vi "HEWH Draw Initialize All Parameters.vi"(0 "Core HEWH Data Input in":T1 {"Test Patten Setup"."PRAT/RLT Sequence"."Time" format="%<%H:%M:%S>t"; "Test Patten Setup"."Total Gallons Schedule" format="%.2f"}, 1 "Station Draw Info":T3 {"Time" format="%<%H:%M:%S>t"}, 2 "Skip Draw":bool, 3 "Skip Purge":bool, 5 "Error In":errorcluster, 7 "K-Factor (Intellifaucet)":dbl, 9 "Current Cond":T8, 11 "K-Factor (Flow)":dbl, 13 "Intellifaucet Type":string) -> (14 "Core HEWH Data Input out":T1 {"Test Patten Setup"."PRAT/RLT Sequence"."Time" format="%<%H:%M:%S>t"; "Test Patten Setup"."Total Gallons Schedule" format="%.2f"}, 15 "Skip Draw":bool, 16 "Skip Purge":bool, 17 "Skip Valve Setup":bool, 19 "Error Out":errorcluster)   [LabVIEW 2016]
uses:
  Type Definitions/HEWH Special Condition Check.ctl
  Type Definitions/HEWH Output Information.ctl
  Type Definitions/HEWH Draw Pattern Setup.ctl
  Type Definitions/PRAT Test.ctl
  Utility/Save File/File Setup (Public)/Type Definition/Save File HEWH Heating Control Mode.ctl
  Type Definitions/Terminate Draw Conditions.ctl
  Type Definitions/HEWH Start Conditions.ctl
  Type Definitions/Check Special Condtions.ctl
  Type Definitions/HEWH Draw Flag ENUM.ctl
  Type Definitions/HEWH Specific DAQ.ctl
  Type Definitions/HEWH Power Data.ctl
  Type Definitions/HEWH Power Elements.ctl
  Utility/Type Definitions/UTILITY Power Analyzer.ctl
  Type Definitions/HEWH Calc and Calibration.ctl
  Utility/Save File/File Setup (Public)/Type Definition/Save File DOE LabView Program.ctl
  Custom Instrument Control/MW100/Type Definitions/Station ID Selector.ctl
  Range/Type Definitions/RANGE ANSI Rate.ctl
  Utility/Save File/File Setup.lvlib
panel:
  # "Draw Pattern Setup (24 Hour)"
  # "Draw Pattern Setup (24 Hour)"
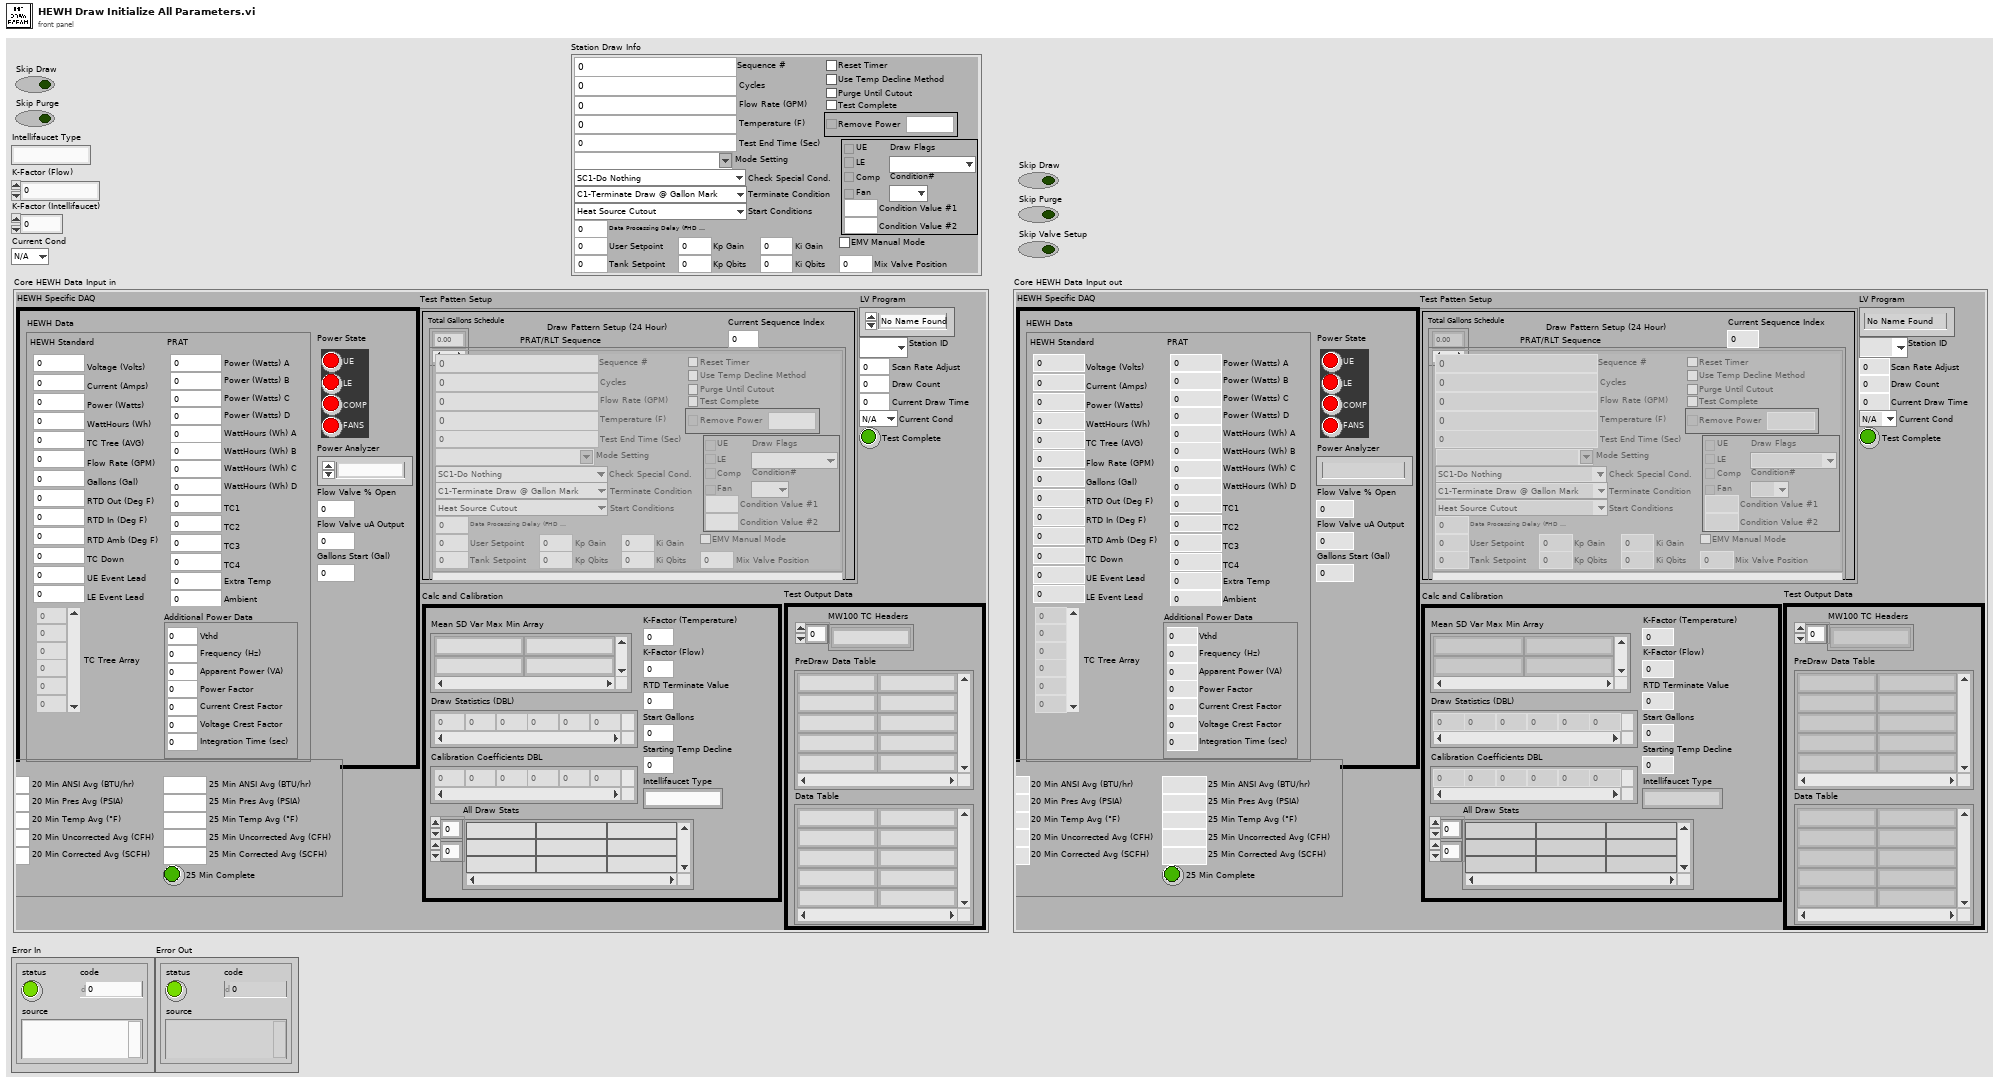
[diagram p1: front panel]
types:
  T1 = typedef "HEWH Output Information.ctl" = cluster{"Scan Rate Adjust":dbl, "Draw Count":i32, "Test Patten Setup":T2, "HEWH Specific DAQ":T10, "Test Output Data":cluster{"PreDraw Data Table":string[][], "Data Table":string[][], "MW100 TC Headers":string[]}, "Calc and Calibration":T14, "Current Draw Time":dbl, "LV Program":T15, "Station ID":T16, "Current Cond":T8, "Test Complete":bool, "ANSI Rate":T17}
  T2 = typedef "HEWH Draw Pattern Setup.ctl" = cluster{"Total Gallons Schedule":dbl[], "PRAT/RLT Sequence":T3[], "Current Sequence Index":i32}
  T3 = typedef "PRAT Test.ctl" = cluster{"Sequence #":dbl, "Cycles":i32, "Mode Setting":T4, "Flow Rate (GPM)":dbl, "Temperature (F)":dbl, "Reset Timer":bool, "Use Temp Decline Method":bool, "Terminate Condition":T5, "Condition Value #1":dbl, "UE":bool, "LE":bool, "Comp":bool, "Fan":bool, "Test End Time (Sec)":dbl, "Purge Until Cutout":bool, "Start Conditions":T6, "Condition Value #2":dbl, "Remove Power":bool, "Time":dbl, "Check Special Cond.":T7, "Condition#":T8, "Draw Flags":T9, "Data Processing Delay (FHD 15sec, UEF 5 Sec)":dbl, "Test Complete":bool, "User Setpoint":dbl, "Tank Setpoint":dbl, "Kp Gain":dbl, "Kp Qbits":dbl, "Ki Gain":dbl, "Ki Qbits":dbl, "Mix Valve Position":i16, "EMV Manual Mode":bool}
  T4 = typedef "File Setup.lvlib/Save File HEWH Heating Control Mode.ctl" = string
  T5 = typedef "Terminate Draw Conditions.ctl" = enum16{"C1-Terminate Draw @ Gallon Mark", "C2-Special Last Draw (HU Test)", "C3-RTD Out <=", "C4-Mean Tank Temp <=", "C5-Decrease RTD Out (Deg F)", "C6-Time (Seconds)", "C7-Until Any Heat Source", "C8-Specific Heat Source", "C9-Do Nothing"}
  T6 = typedef "HEWH Start Conditions.ctl" = enum16{"Heat Source Cutout", "At Time (Seconds)", "Every X (Seconds)", "T2 >= X° Below Setpoint", "Seconds From Complete", "Wait for LE & Comp Cutout", "Wait for Comp Cutout", "Wait for LE Cutout", "Wait for UE Cutout"}
  T7 = typedef "Check Special Condtions.ctl" = enum16{"SC1-Do Nothing", "SC2-Check Heat Source (On-C2/Off-C1)", "SC3-Check Skip Condition", "SC4-Check Heat Source ON/Fail"}
  T8 = typedef "HEWH Special Condition Check.ctl" = enum16{"N/A", "C1", "C2", "Reset/Fail", "Skip Draw Sequence"}
  T9 = typedef "HEWH Draw Flag ENUM.ctl" = enum16{"N/A", "None(0)", "Sml(1)", "Med(2)", "SmlMed(3)", "Lrg(4)", "SmlLrg(5)", "MedLrg(6)", "SmlMedLrg(7)"}
  T10 = typedef "HEWH Specific DAQ.ctl" = cluster{"HEWH Data":T11, "Flow Valve % Open":dbl, "Power State":T12, "Power Analyzer":T13, "Flow Valve uA Output":i32, "Gallons Start (Gal)":dbl}
  T11 = typedef "HEWH Power Data.ctl" = cluster{"HEWH Standard":cluster{"Voltage (Volts)":dbl, "Current (Amps)":dbl, "Power (Watts)":dbl, "WattHours (Wh)":dbl, "TC Tree (AVG)":dbl, "Flow Rate (GPM)":dbl, "Gallons (Gal)":dbl, "RTD Out (Deg F)":dbl, "RTD In (Deg F)":dbl, "RTD Amb (Deg F)":dbl, "TC Down":dbl, "UE Event Lead":i32, "LE Event Lead":i32, "TC Tree Array":dbl[]}, "PRAT":cluster{"Power (Watts) A":dbl, "Power (Watts) B":dbl, "Power (Watts) C":dbl, "Power (Watts) D":dbl, "TC1":dbl, "TC2":dbl, "TC3":dbl, "TC4":dbl, "WattHours (Wh) A":dbl, "WattHours (Wh) B":dbl, "WattHours (Wh) C":dbl, "WattHours (Wh) D":dbl, "Ambient":dbl, "Extra Temp":dbl}, "Additional Power Data":cluster{"Vthd":dbl, "Frequency (Hz)":dbl, "Apparent Power (VA)":dbl, "Power Factor":dbl, "Current Crest Factor":dbl, "Voltage Crest Factor":dbl, "Integration Time (sec)":dbl}}
  T12 = typedef "HEWH Power Elements.ctl" = cluster{"UE":bool, "LE":bool, "COMP":bool, "FANS":bool}
  T13 = typedef "UTILITY Power Analyzer.ctl" = enum16{"", "APLUS", "WT210", "WT500", "WT300", "OSI", "Debug", "WT230", "WT300_1", "WT300_2"}
  T14 = typedef "HEWH Calc and Calibration.ctl" = cluster{"Mean SD Var Max Min Array":string[][], "Draw Statistics (DBL)":dbl[][], "Calibration Coefficients DBL":dbl[][], "Start Gallons":dbl, "Starting Temp Decline":dbl, "K-Factor (Temperature)":dbl, "All Draw Stats":string[][], "RTD Terminate Value":dbl, "K-Factor (Flow)":dbl, "Intellifaucet Type":string}
  T15 = typedef "File Setup.lvlib/Save File DOE LabView Program.ctl" = enum16{"No Name Found", "DOE Stand", "Dishwasher Kitchen", "Portable Stand", "HEWH", "Dryer", "Dryer WILT", "HCC", "PRAT", "HEWH RLT", "Refrigeration"}
  T16 = typedef "Station ID Selector.ctl" = enum16{"", "A", "B", "C", "D", "Global"}
  T17 = typedef "RANGE ANSI Rate.ctl" = cluster{"Array 1":dbl[], "Array 3":dbl[], "Array 2":dbl[], "Start ANSI":bool, "ANSI Start Time":dbl, "Restart ANSI":bool, "15 Min ANSI Avg (BTU/hr)":dbl, "20 Min ANSI Avg (BTU/hr)":dbl, "25 Min ANSI Avg (BTU/hr)":dbl, "Absolute Pressure":dbl, "Gas Temperature":dbl, "Volumetric Flow Rate":dbl, "Mass Flow Rate":dbl, "Array 4":dbl[], "Array 5":dbl[], "Gas Rate":dbl, "15 Min Pres Avg (PSIA)":dbl, "20 Min Pres Avg (PSIA)":dbl, "25 Min Pres Avg (PSIA)":dbl, "15 Min Temp Avg (°F) ":dbl, "20 Min Temp Avg (°F)":dbl, "25 Min Temp Avg (°F)":dbl, "15 Min Uncorrected Avg (CFH)":dbl, "20 Min Uncorrected Avg (CFH)":dbl, "25 Min Uncorrected Avg (CFH)":dbl, "15 Min Corrected Avg (SCFH)":dbl, "20 Min Corrected Avg (SCFH)":dbl, "25 Min Corrected Avg (SCFH)":dbl, "15 Min Complete":bool, "20 Min Complete":bool, "25 Min Complete":bool}
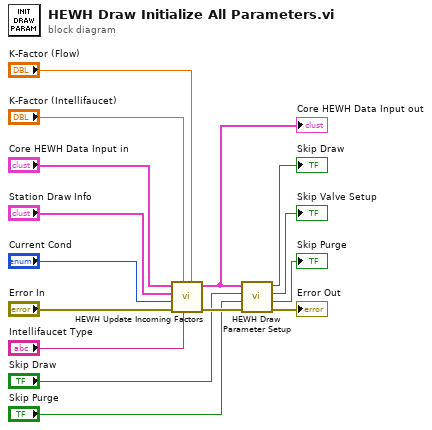
[diagram p0: block diagram]
diagram:
  n1 = call "HEWH Update Incoming Factors.vi"("K-Factor (Flow)"="K-Factor (Flow)", "Intellifaucet Type"="Intellifaucet Type", "K-Factor (Intellifaucet)"="K-Factor (Intellifaucet)", "Error In"="Error In", "Current Cond"="Current Cond", "Station Draw Info"="Station Draw Info", "Core HEWH Data Input in in"="Core HEWH Data Input in") -> ("Error Out"=w7:errorcluster, "Core HEWH Data Input out"=w3:T1)  [unwired: 3 in]
  "Core HEWH Data Input out" <- w3
  n2 = call "HEWH Draw Parameter Setup.vi"("Error In"=w7, "Skip Purge in"="Skip Purge", "Skip Draw in"="Skip Draw", "Core HEWH Data Input in"=w3) -> ("Error Out"=→"Error Out":errorcluster, "Skip Purge out"=→"Skip Purge":bool, "Skip Valve Setup"=→"Skip Valve Setup":bool, "Skip Draw out"=→"Skip Draw":bool)  [unwired: 4 in]
